vi "TSL_Sample.vi"() -> ()   [LabVIEW 2017]
uses:
  D:/test/FULLband-sts/Fullband_Sample/DLL/InstrumentDLL.dll
  DLL/InstrumentDLL.dll
  <vilib>/Utility/miscctls.llb/LVStringsAndValuesArrayTypeDef_DBL.ctl
  <vilib>/Utility/file.llb/Write To Spreadsheet File (DBL).vi
panel:
  in  "选项卡控件":T1(tab)
  in  "btnUsb_resouce":bool
  out "USB device number":string
  in  "Usb resouce":u16(ring)
  out "SweepSpeed Range":string
  in  "Port number":dbl
  in  "Target":enum32{"rdo550", "rdo570"}(radio)
  in  "btnSplit":bool
  out "GPIB Address":dbl
  out "GPIB Boad":dbl
  in  "btnGet_Visa":bool
  in  "Visa String":u16(ring)
  in  "Communication":T2(radio)
  in  "Terminator":enum32{"rdiCr", "rdiLf", "rdiCrLf"}(radio)
  out "Serial":string
  out "Product":string
  out "F/ W Vesion":string
  out "Frequency range":string
  out "Wavelength range":string
  out "APC Limit(dBm)":string
  out "APC Limit(mW)":string
  out "ATT range":string
  in  "Btn_Connect":bool
  in  "Btn_DisConnect":bool
  in  "Address/Device number":string
  out "unit":enum16{"dBm", "mW", ""}(ring)=enum.""
  out "txtshutter":enum16{"Shutter_Open", "Shutter_Close", ""}(ring)=enum.""
  out "status":enum16{"Coh_OFF", "Coh_ON", ""}(ring)=enum.""
  out "mode":enum16{"ACC", "APC", ""}(ring)=enum.""
  out "txtlds":enum16{"LD_OFF", "LD_ON", ""}(ring)=enum.""
  out "LAN Port number":i32
  in  "Get LAN Port":bool
  out "IP Address":string
  in  "Get IP Address":bool
  in  "BtnLD_ON":bool
  in  "BtnLD_OFF":bool
  in  "BtnCoh_ON":bool
  in  "BtnCoh_OFF":bool
  in  "BtnShutter_Open":bool
  in  "BtnShutter_Close":bool
  in  "BtnAPC":bool
  in  "BtnACC":bool
  in  "BtndBm":bool
  in  "BtnmW":bool
  in  "Setting ATT":dbl
  in  "Btn_SetATT":bool
  in  "Setting Power":dbl
  in  "Btn_SetdBm":bool
  in  "Btn_SetmW":bool
  in  "Btn_GetLD":bool
  in  "BtnPower_mode":bool
  in  "BtnCoh_Status":bool
  in  "BtnShutter_Status":bool
  in  "BtnUnit":bool
  out "txtreadatt":dbl
  in  "BtnAtt_value":bool
  out "txtreadpow":dbl
  in  "BtnPower_dBm":bool
  out "txtreadmw":dbl
  in  "BtnPower_mW":bool
  out "txtreadmoni":dbl
  in  "Btnmonitor_dBm":bool
  out "txtradmoni_mw":dbl
  in  "Btnmonitor_mW":bool
  in  "txtsetwave":dbl
  in  "Btn_SetWavelength":bool
  in  "txtsetfreq":dbl
  in  "Btn_SetFrequency":bool
  in  "txtsetft":dbl
  in  "Btn_SetFinetuning":bool
  in  "Btn_Wavelength":bool
  in  "Btn_Frequency":bool
  in  "Btn_Fine":bool
  out "txtwave":dbl
  out "txtfreq":dbl
  out "txtfine":dbl
  out "txtbusy":string
  in  "Btn_Busy":bool
  in  "Wait time(msec)":i32
  in  "Btn_Stangby":bool
  out "txttsl_err":string
  in  "Btn_error":bool
  out "Start mode":enum16{"Normal", "WaitingforTrigger", ""}(ring)=enum.""
  out "Trigger output":enum16{"None", "Stop", "Start", "Step", ""}(ring)=enum.""
  out "Trigger input":enum16{"Disable", "Enable", ""}(ring)=enum.""
  out "Sweep Mode":T3(ring)=enum.""
  out "txtg_sweep_su":T4(ring)=enum."Returning"
  out "Trigger Source":enum16{"Wavelength", "Time", ""}(ring)=enum.""
  in  "Speed(570)":u16(ring) caption="Speed(nm/sec)" items=["1"=1, "2"=2, "5"=5, "10"=10, "20"=20, "50"=50, "100"=100, "200"=200]
  in  "Speed":u16(ring)
  in  "Get speed table":bool
  in  "cmbTrigger_Source":enum16{"Wavelength", "Time", ""}(ring) caption="Trigger Source(570)"
  in  "txtstart":dbl caption="Start wavelength"
  in  "Btn_SetWavelength_Parameters":bool
  in  "txtstop":dbl caption="Stop wavelength"
  in  "txtstep":dbl=0.1 caption="Trigger/wave step"
  in  "txtspeed(550)":dbl caption="Speed(nm/sec)"
  in  "Btn_Other":bool
  in  "txtdelay":dbl caption="Delay time(sec)"
  in  "txtcycle":i32=1 caption="cycle"
  in  "cmbsm":T5(ring) caption="Sweep Mode"
  in  "cmbst_mod":enum16{"Disable", "Enable"}(ring) caption="Trigger input"
  in  "cmbtout":enum16{"None", "Stop", "Start", "Step"}(ring) caption="Trigger output"
  in  "cmbtin":enum16{"Normal", "Waiting for Trigger"}(ring) caption="Start mode"
  out "Start wavelength":dbl
  out "Stop wavelength":dbl
  out "Wavelength step":dbl
  out "Trigger step":dbl
  out "Speed(nm/sec)":dbl
  out "Delay time(sec)":dbl
  out "cycle":i32
  in  "BtnGet_setting":bool
  in  "Status":u16(ring) items=["Standby", "Running", "Pauseing", "WaitingforTrigger", "Returning"]
  in  "Wait time(msec)":i32
  in  "Btn_Waiting":bool
  in  "Btn_Status":bool
  in  "Btn_Minstep":bool
  in  "txtspeed":dbl=100.0
  out "txtcurrentc":i32
  in  "Btn_Current":bool
  in  "Btn_Start":bool
  in  "Btn_Stop":bool
  in  "Btn_SoftwareTrigger":bool
  in  "Btn_Pause":bool
  in  "Btn_ReStart":bool
  in  "Btn_GetLogg":bool
  out "TSL":refnum<k24>
  # "0. Connect Tool"
  # "1. Connect"
  # "Information"
  # "Power Control"
  # "Power status"
  # "Wavelength Control"
  # "Wavelength Status"
  # "Common Function"
  # "Sweep Setting"
  # "Other"
  # "Wavelength parameters"
  # "Other parameters"
  # "Sweep Speed(nm/s)"
  # "Sweep setting status"
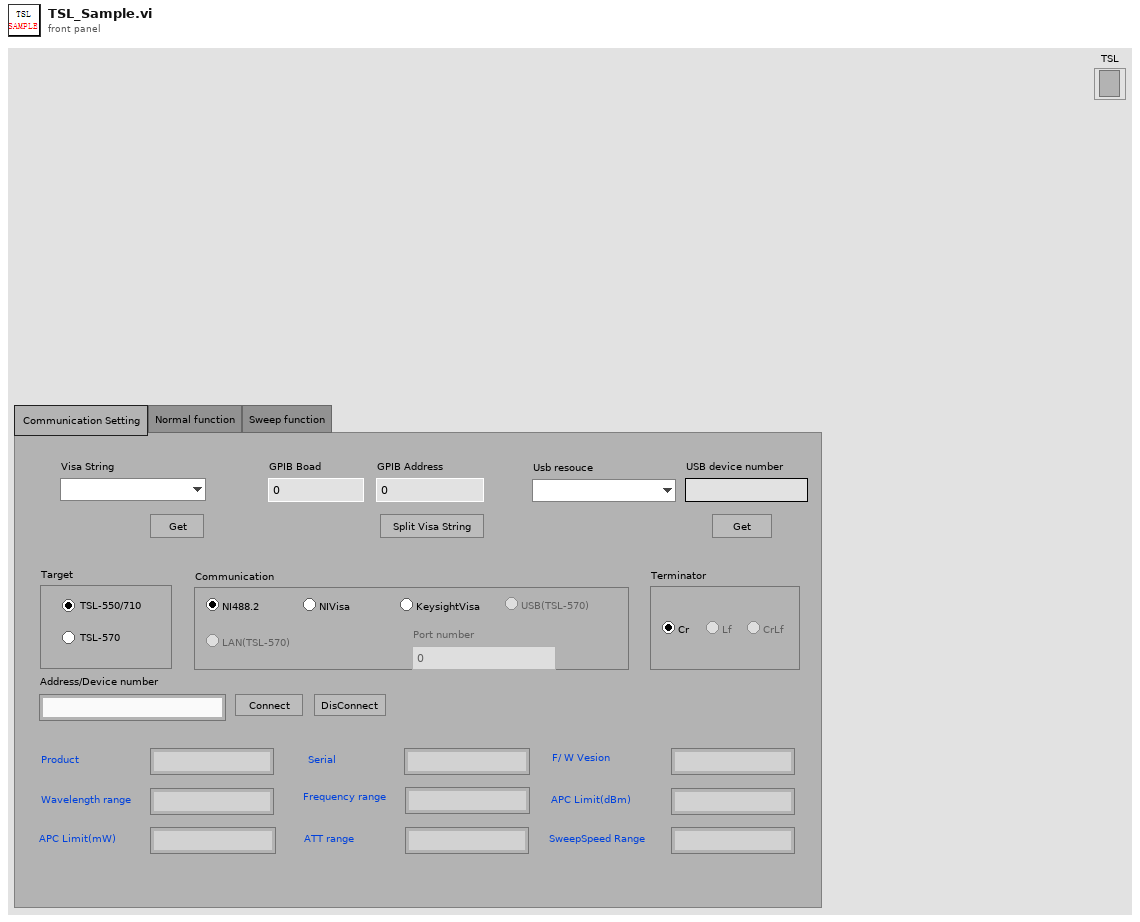
[diagram p1: front panel]
types:
  T1 = enum32{"Communication Setting ", "Normal function", "Sweep function"}
  T2 = enum32{"rdiNI488", "rdiNIvisa", "rdikysightvisa", "rdiUSB", "rdiLAN"}
  T3 = enum16{"Step_Oneway", "Continuous_Oneway", "Step_Twoway", "Continuous_Twoway", ""}
  T4 = enum16{"Standby", "Running", "Pausing", "WaitingforTrigger", "Returning"}
  T5 = enum16{"Step one way", "Continuous one way", "Step round trip", "Continuous round trip"}
  T6 = enum16{"Standby", "Running", "Pausing", "WaitingforTrigger", "Returning", ""}
  T7 = enum8{"Enabled", "Disabled", "Disabled and Grayed Out"}
  T8 = typedef "LVStringsAndValuesArrayTypeDef_DBL.ctl" = cluster{"String":string, "Value":dbl}[]
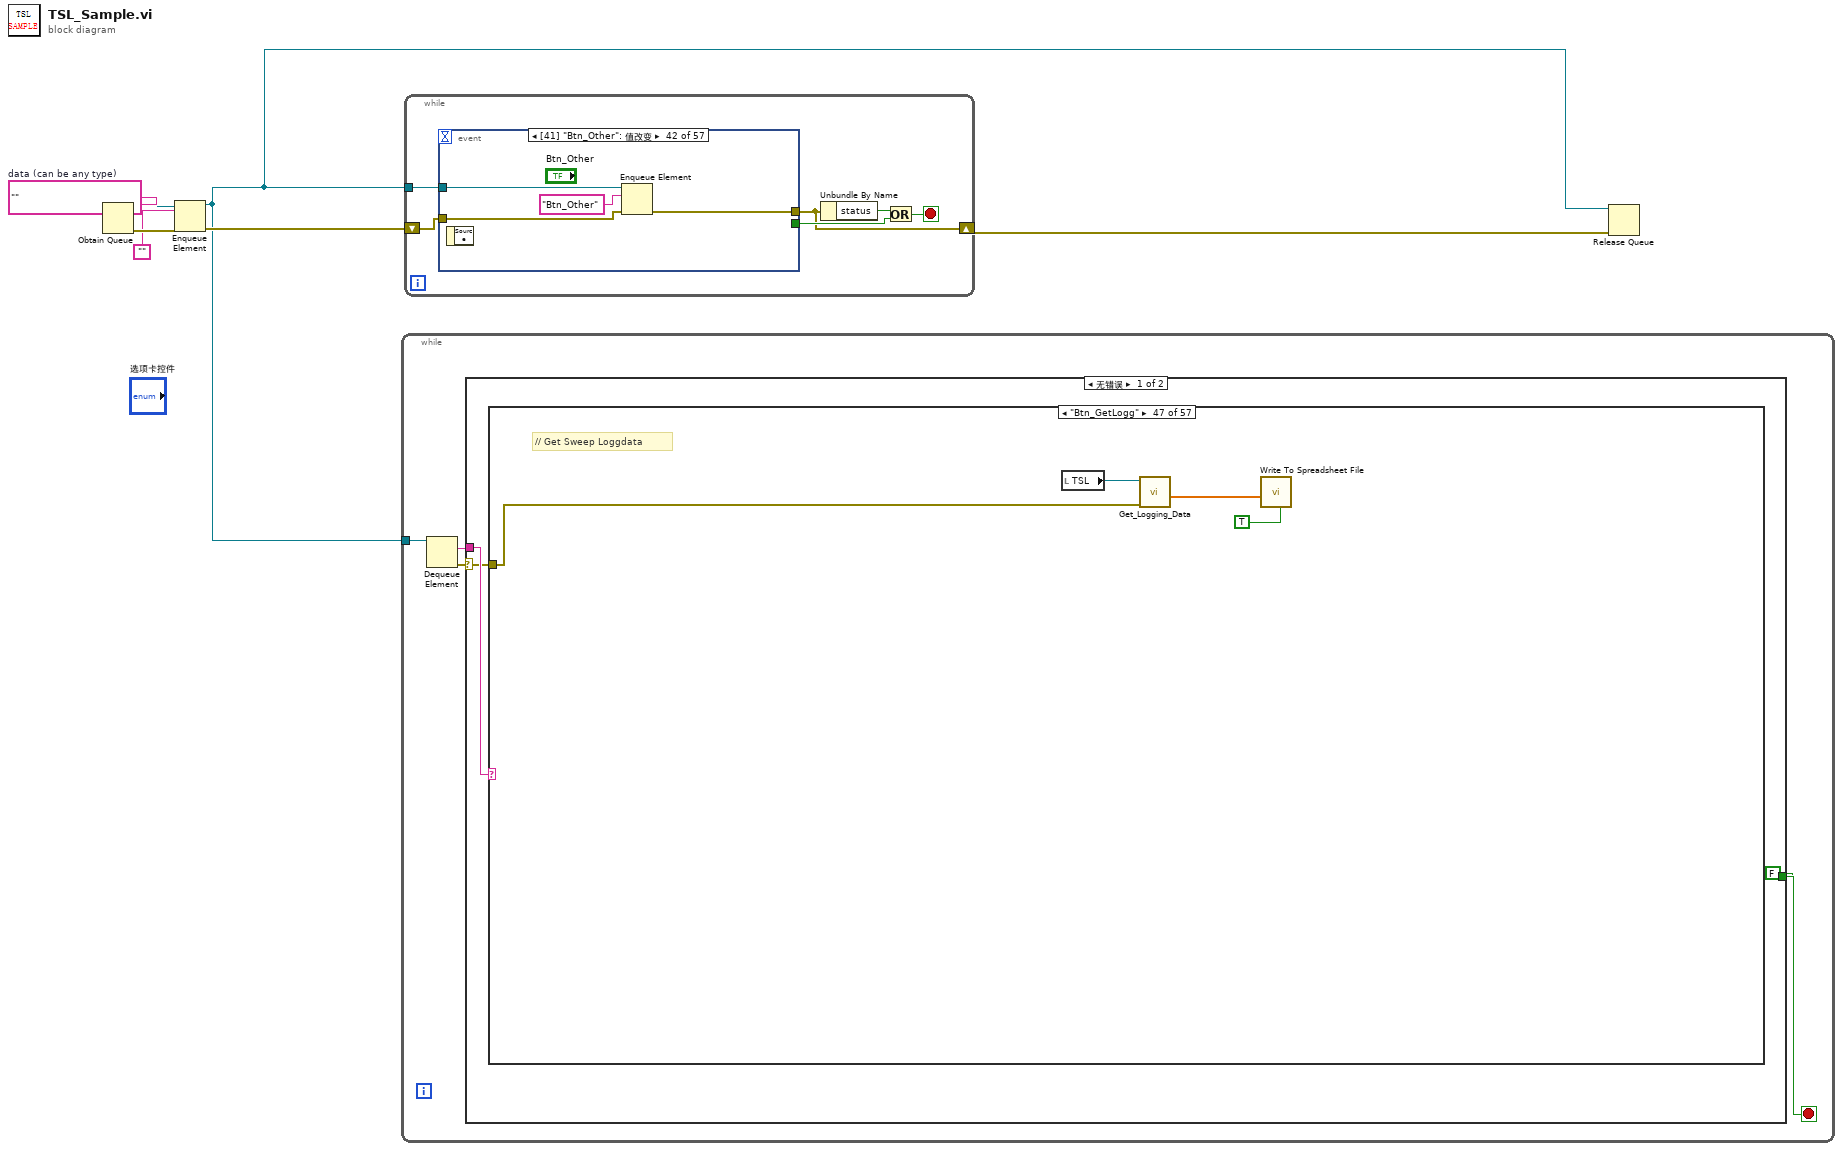
[diagram p0: block diagram]
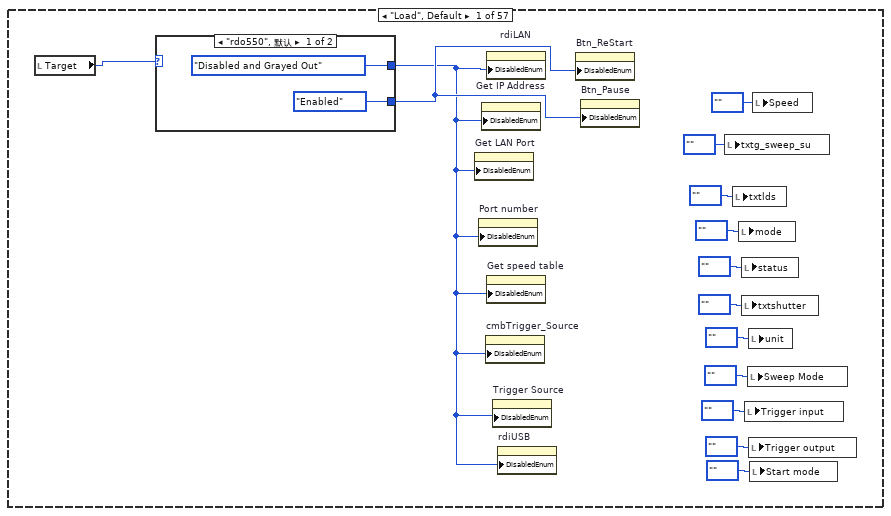
[diagram p2: hidden frame]
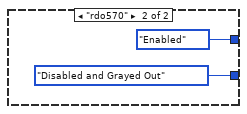
[diagram p3: hidden frame]
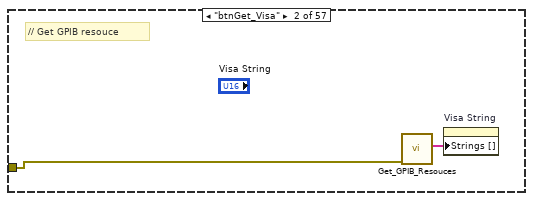
[diagram p4: hidden frame]
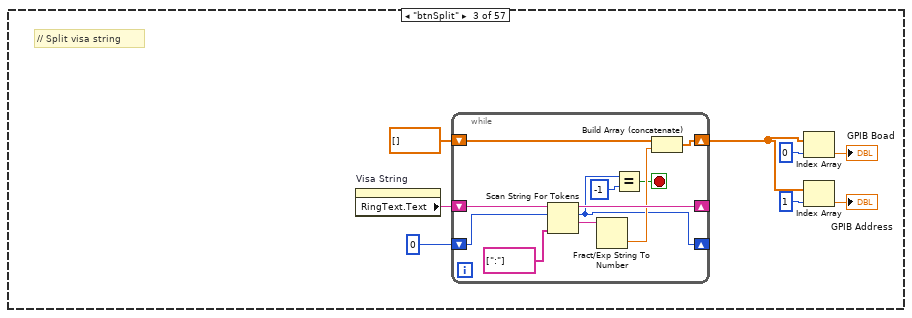
[diagram p5: hidden frame]
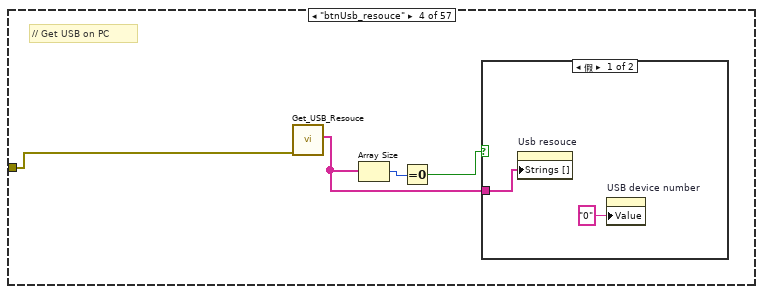
[diagram p6: hidden frame]
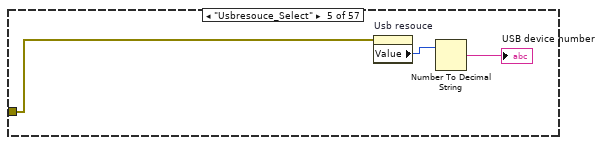
[diagram p8: hidden frame]
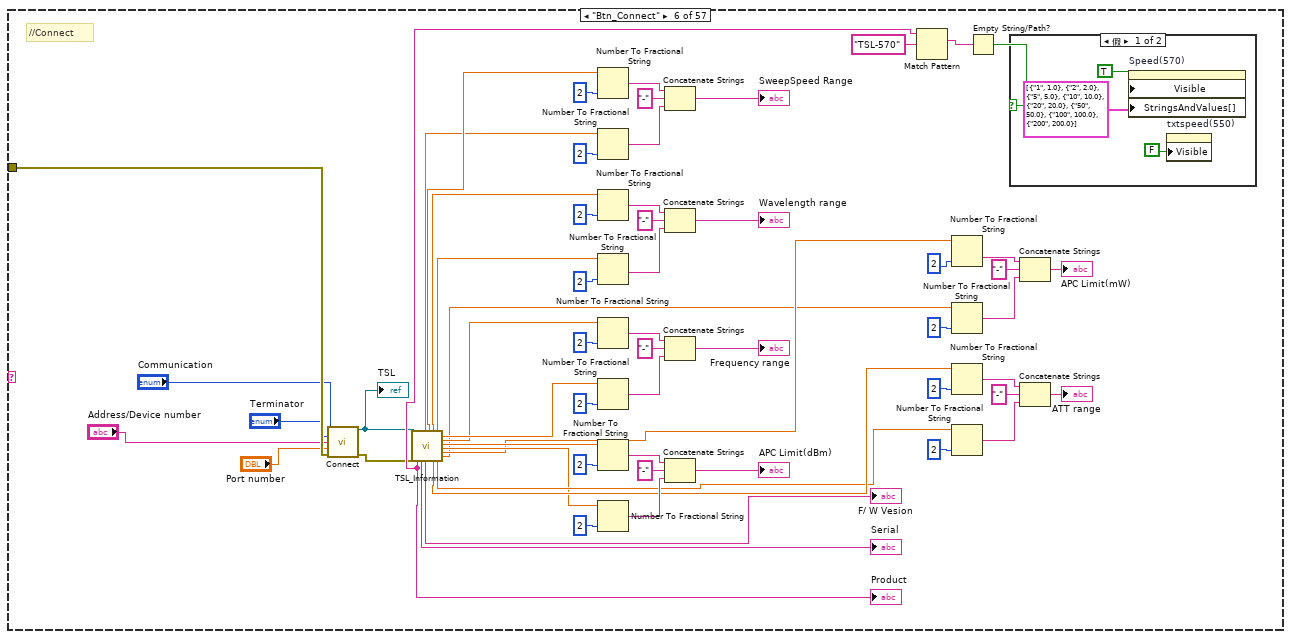
[diagram p9: hidden frame]
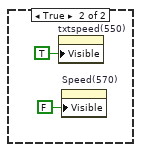
[diagram p10: hidden frame]
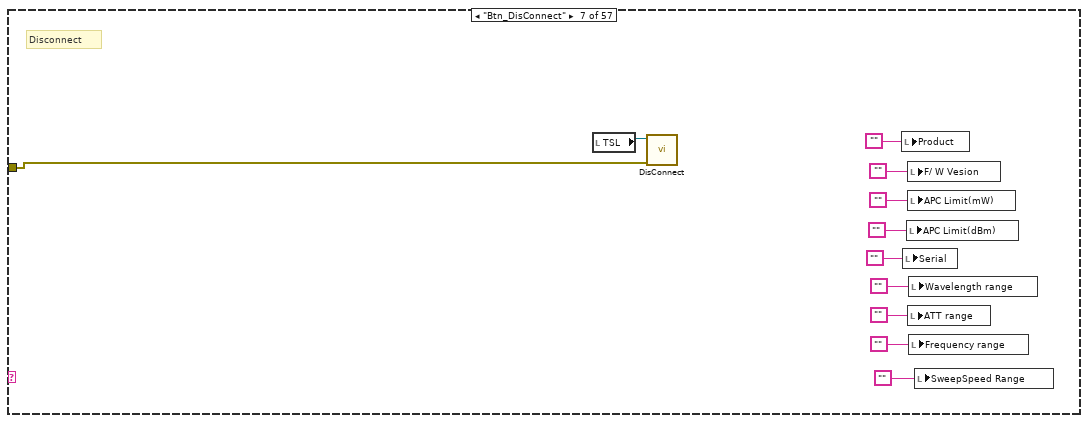
[diagram p11: hidden frame]
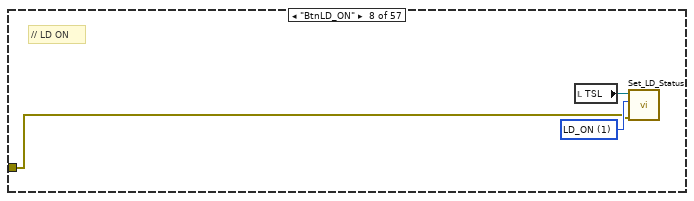
[diagram p12: hidden frame]
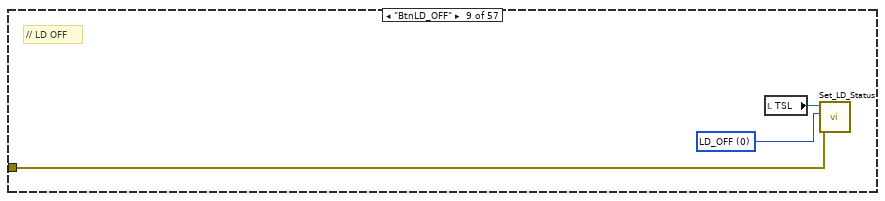
[diagram p13: hidden frame]
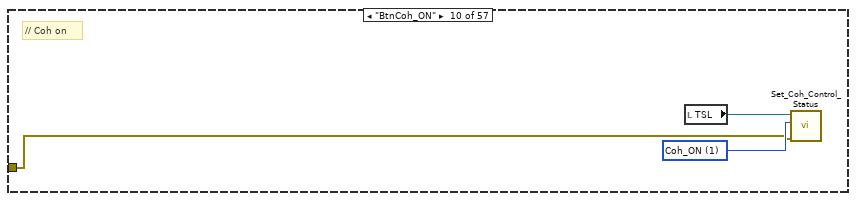
[diagram p14: hidden frame]
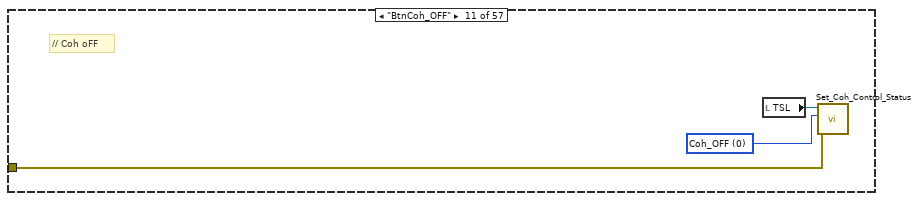
[diagram p15: hidden frame]
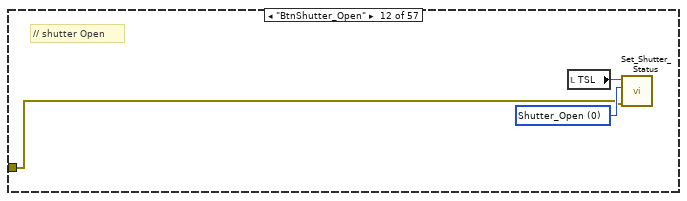
[diagram p16: hidden frame]
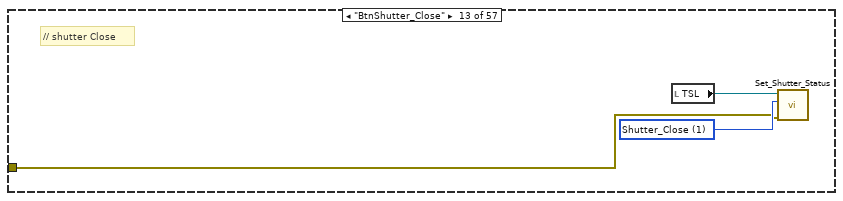
[diagram p17: hidden frame]
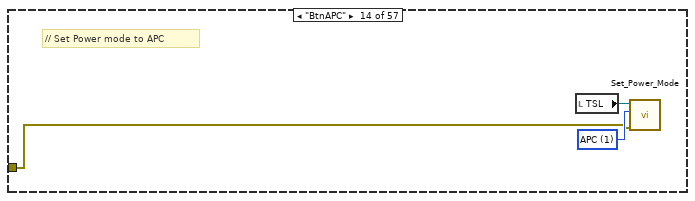
[diagram p18: hidden frame]
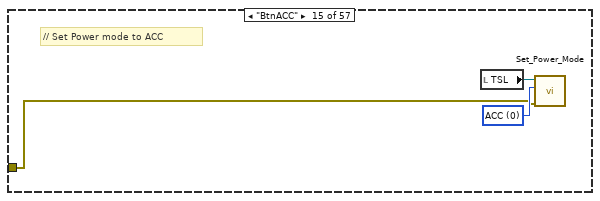
[diagram p19: hidden frame]
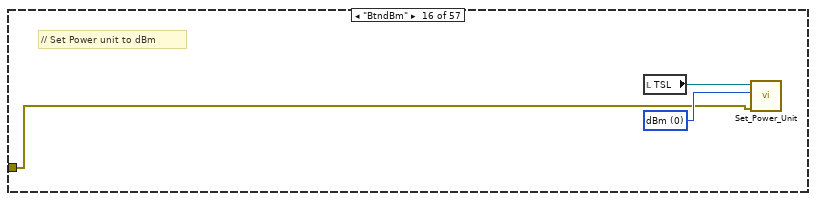
[diagram p20: hidden frame]
diagram:
  w4 = ""  # data (can be any type)
  n1 = Obtain Queue(element data type=w4) -> (queue out=w3:refnum<queue>, error out=w7:errorcluster)  [unwired: 4 in, 1 out]
  n2 = Enqueue Element(queue=w3, element="", error in (no error)=w7) -> (queue out=w1:refnum<queue>, error out=w6:errorcluster)  [unwired: 1 in, 1 out]
  n3 = while {
    tunnel: w1 -> [w11]
    stop <- w8 stop-if-true
    n4 = Dequeue Element(queue=w11) -> (element=w9:string, error out=w10:errorcluster)  [unwired: 2 in, 2 out]
    n5 = case shown="无错误" w10 {
      selector: w10 -> [w12 _]
      tunnel: w9 -> [w14 _]
      tunnel: [FALSE TRUE] -> w8
      frame No Error {
        n6 = case shown="\"Btn_GetLogg\"" w14 {
          tunnel: w12 -> [_ w33 _ w54 w62 w68 w129 w140 w143 w146 w149 w152 w155 w158 w161 w164 w167 w170 w173 w177 w179 w182 w185 w188 w191 w194 w197 w202 w215 _ w234 w238 w240 w244 w247 w250 w252 w255 w258 w261 w264 w267 w276 w300 w336 w351 w354 w357 w360 w368 w370 w372 w374 w378 w380 w383 _]
          frame "Load", Default {
            n7 = local read "Target"() -> (w27:enum32{"rdo550", "rdo570"})
            n8 = case shown="\"rdo550\", 默认" w27 {
              tunnel: [T7."Disabled and Grayed Out" ("禁用") T7."Enabled" ("禁用")] -> w26
              tunnel: [T7."Enabled" ("禁用") T7."Disabled and Grayed Out" ("禁用")] -> w28
              frame "rdo550", Default {
              }
              frame "rdo570" {
              }
            }
            n9 = property on="Get LAN Port" class="Bool"("DisabledEnum"=w26) -> ()  [unwired: 2 in, 2 out]
            n10 = property on="Port number" class="DigNum (严格)"("DisabledEnum"=w26) -> ()  [unwired: 2 in, 2 out]
            n11 = property on="Get IP Address" class="Bool"("DisabledEnum"=w26) -> ()  [unwired: 2 in, 2 out]
            n12 = property on="cmbTrigger_Source" class="Enum (严格)"("DisabledEnum"=w26) -> ()  [unwired: 2 in, 2 out]
            n13 = property on="rdiLAN" class="Bool (严格)"("DisabledEnum"=w26) -> ()  [unwired: 2 in, 2 out]
            n14 = property on="Get speed table" class="Bool"("DisabledEnum"=w26) -> ()  [unwired: 2 in, 2 out]
            n15 = property on="Trigger Source" class="Enum (严格)"("DisabledEnum"=w26) -> ()  [unwired: 2 in, 2 out]
            n16 = property on="rdiUSB" class="Bool (严格)"("DisabledEnum"=w26) -> ()  [unwired: 2 in, 2 out]
            n17 = property on="Btn_ReStart" class="Bool"("DisabledEnum"=w28) -> ()  [unwired: 2 in, 2 out]
            n18 = property on="Btn_Pause" class="Bool"("DisabledEnum"=w28) -> ()  [unwired: 2 in, 2 out]
            n19 = local write "txtg_sweep_su"(T6."" ("txtg_sweep_su")) -> ()
            n20 = local write "txtlds"(enum16{"LD_OFF", "LD_ON", ""}."" ("txtlds")) -> ()
            n21 = local write "mode"(enum16{"ACC", "APC", ""}."" ("mode")) -> ()
            n22 = local write "status"(enum16{"Coh_OFF", "Coh_ON", ""}."" ("status")) -> ()
            n23 = local write "txtshutter"(enum16{"Shutter_Open", "Shutter_Close", ""}."" ("txtshutter")) -> ()
            n24 = local write "Trigger input"(enum16{"Disable", "Enable", ""}."" ("Trigger input")) -> ()
            n25 = local write "Sweep Mode"(T3."" ("Sweep Mode")) -> ()
            n26 = local write "unit"(enum16{"dBm", "mW", ""}."" ("unit")) -> ()
            n27 = local write "Trigger output"(enum16{"None", "Stop", "Start", "Step", ""}."" ("Trigger output")) -> ()
            n28 = local write "Start mode"(enum16{"Normal", "WaitingforTrigger", ""}."" ("Start mode")) -> ()
            n29 = local write "Speed"(enum16{""}."" ("Speed")) -> ()
          }
          frame "btnGet_Visa" {
            # "// Get GPIB resouce"
            n30 = call "Get_GPIB_Resouces.vi"("error in (no error)"=w33) -> ("Get_GPIB_Resources"=w34:string[])  [unwired: 8 in, 2 out]
            n31 = property on="Visa String" class="Ring (严格)"("Strings []"=w34) -> ()  [unwired: 2 in, 2 out]
          }
          frame "btnSplit" {
            # "// Split visa string"
            n32 = property on="Visa String" class="Ring (严格)"() -> ("RingText.Text"=w38:string)  [unwired: 2 in, 2 out]
            n33 = while {
              shift-right: [w52] -> _
              shift-left: w38 -> [w53]
              shift-right: [w48] -> w40
              shift-left: dbl[] [] ("数组") -> [w49]
              shift-right: [w43] -> _
              shift-left: 0 ("偏移量") -> [w44]
              stop <- w46 stop-if-true
              n34 = Scan String For Tokens(6:string[] [":"] ("分隔符(\\s,\\t,\\r,\\n)"), 8:w44, 9:w53) -> (1:w51:string, 2:w43:i32, 3:w52:string)  [unwired: 3 in, 1 out]
              n35 = Fract/Exp String To Number(string=w51) -> (number=w50:dbl)  [unwired: 3 in, 1 out]
              n36 = Equal?(x=w43, y=-1) -> (x = y?=w46:bool)
              n37 = Build Array (concatenate)(w49, w50) -> (w48:dbl[])
            }
            n38 = Index Array(array=w40, index=0 ("索引")) -> (element=→"GPIB Boad":dbl)
            n39 = Index Array(array=w40, index=1 ("索引")) -> (element=→"GPIB Address":dbl)
          }
          frame "btnUsb_resouce" {
            # "// Get USB on PC"
            n40 = call "Get_USB_Resouce.vi"("error in (no error)"=w54) -> ("Get_USB_Resouce"=w55:string[])  [unwired: 8 in, 2 out]
            n41 = Array Size(array=w55) -> (size(s)=w57:i32)
            n42 = Equal To 0?(x=w57) -> (x = 0?=w56:bool)
            n43 = case shown="假" w56 {
              tunnel: w55 -> [w59 _]
              frame False {
                n44 = property on="Usb resouce" class="Ring (严格)"("Strings []"=w59) -> ()  [unwired: 2 in, 2 out]
                n45 = property on="USB device number" class="Str"("Value"="0" ("USB device number")) -> ()  [unwired: 2 in, 2 out]
              }
              frame True {
              }
            }
          }
          frame "Usbresouce_Select" {
            n46 = property on="Usb resouce" class="Ring (严格)"(error in=w62) -> ("Value"=w61:u16)  [unwired: 1 in, 2 out]
            n47 = Number To Decimal String(number=w61) -> (decimal integer string=→"USB device number":string)  [unwired: 1 in]
          }
          frame "Btn_Connect" {
            # "//Connect"
            n48 = call "Connect.vi"("Communication"="Communication", "Terminator"="Terminator", "Address/Device number"="Address/Device number", "Port"="Port number", "error in (no error)"=w68) -> ("Reference out"=w69:refnum<k24>, "error out"=w67:errorcluster)  [unwired: 9 in]
            "TSL" <- w69
            n49 = call "TSL_Information.vi"(".NET Reference in"=w69, "error in (no error)"=w67) -> ("ProductName"=w70:string, "SerialNumber"=→"Serial":string, "MaximumSpeed"=w79:dbl, "FWversion"=→"F/ W Vesion":string, "MinimumSpeed"=w80:dbl, "MinimunWavelength"=w78:dbl, "MinimumATTValue"=w82:dbl, "MaximumWavelength"=w77:dbl, "MaximumATTValue"=w81:dbl, "MaximumFrequency"=w76:dbl, "MinimunFrequency"=w75:dbl, "MinimumAPCPower_dBm"=w74:dbl, "MaximumAPCPower_dBm"=w73:dbl, "MinimumAPCPower_mW"=w72:dbl, "MaximumAPCPower_mW"=w71:dbl)  [unwired: 9 in, 2 out]
            "Product" <- w70
            n50 = Number To Fractional String(number=w80, precision (6)=i16 2 ("精度(6)")) -> (F-format string=w92:string)  [unwired: 2 in]
            n51 = Number To Fractional String(number=w79, precision (6)=i16 2 ("精度(6)")) -> (F-format string=w91:string)  [unwired: 2 in]
            n52 = Number To Fractional String(number=w78, precision (6)=i16 2 ("精度(6)")) -> (F-format string=w118:string)  [unwired: 2 in]
            n53 = Number To Fractional String(number=w77, precision (6)=i16 2 ("精度(6)")) -> (F-format string=w119:string)  [unwired: 2 in]
            n54 = Number To Fractional String(number=w75, precision (6)=i16 2 ("精度(6)")) -> (F-format string=w123:string)  [unwired: 2 in]
            n55 = Number To Fractional String(number=w76, precision (6)=i16 2 ("精度(6)")) -> (F-format string=w122:string)  [unwired: 2 in]
            n56 = Number To Fractional String(number=w74, precision (6)=i16 2 ("精度(6)")) -> (F-format string=w114:string)  [unwired: 2 in]
            n57 = Number To Fractional String(number=w73, precision (6)=i16 2 ("精度(6)")) -> (F-format string=w113:string)  [unwired: 2 in]
            n58 = Concatenate Strings(w92, "-" ("字符串"), w91) -> (→"SweepSpeed Range":string)
            n59 = Concatenate Strings(w118, "-" ("字符串"), w119) -> (→"Wavelength range":string)
            n60 = Concatenate Strings(w123, "-" ("字符串"), w122) -> (→"Frequency range":string)
            n61 = Concatenate Strings(w114, "-" ("字符串"), w113) -> (→"APC Limit(dBm)":string)
            n62 = Match Pattern(string=w70, regular expression="TSL-570" ("正则表达式")) -> (match substring=w86:string)  [unwired: 1 in, 3 out]
            n63 = Number To Fractional String(number=w72, precision (6)=i16 2 ("精度(6)")) -> (F-format string=w111:string)  [unwired: 2 in]
            n64 = Number To Fractional String(number=w71, precision (6)=i16 2 ("精度(6)")) -> (F-format string=w110:string)  [unwired: 2 in]
            n65 = Number To Fractional String(number=w82, precision (6)=i16 2 ("精度(6)")) -> (F-format string=w116:string)  [unwired: 2 in]
            n66 = Number To Fractional String(number=w81, precision (6)=i16 2 ("精度(6)")) -> (F-format string=w115:string)  [unwired: 2 in]
            n67 = Empty String/Path?(string/path=w86) -> (empty?=w85:bool)
            n68 = case shown="假" w85 {
              frame False {
                n69 = property on="Speed(570)" class="Ring (严格)"("Visible"=TRUE ("可见"), "StringsAndValues[]"=T8 [{"String"="1", "Value"=1.0}, {"String"="2", "Value"=2.0}, {"String"="5", "Value"=5.0}, {"String"="10", "Value"=10.0}, {"String"="20", "Value"=20.0}, {"String"="50", "Value"=50.0}, {"String"="100", "Value"=100.0}, {"String"="200", "Value"=200.0}] ("Strings And Values []")) -> ()  [unwired: 2 in, 2 out]
                n70 = property on="txtspeed(550)" class="DigNum (严格)"("Visible"=FALSE ("可见")) -> ()  [unwired: 2 in, 2 out]
              }
              frame True {
                n71 = property on="txtspeed(550)" class="DigNum (严格)"("Visible"=TRUE ("可见")) -> ()  [unwired: 2 in, 2 out]
                n72 = property on="Speed(570)" class="Ring (严格)"("Visible"=FALSE ("可见")) -> ()  [unwired: 2 in, 2 out]
              }
            }
            n73 = Concatenate Strings(w111, "-" ("字符串"), w110) -> (→"APC Limit(mW)":string)
            n74 = Concatenate Strings(w116, "-" ("字符串"), w115) -> (→"ATT range":string)
          }
          frame "Btn_DisConnect" {
            # "Disconnect"
            n75 = local read "TSL"() -> (w131:refnum<k24>)
            n76 = call "DisConnect.vi"("error in (no error)"=w129, ".NET Reference in"=w131) -> ()  [unwired: 4 in, 2 out]
            n77 = local write "Product"("") -> ()
            n78 = local write "Serial"("") -> ()
            n79 = local write "APC Limit(dBm)"("") -> ()
            n80 = local write "F/ W Vesion"("") -> ()
            n81 = local write "APC Limit(mW)"("") -> ()
            n82 = local write "ATT range"("") -> ()
            n83 = local write "Wavelength range"("") -> ()
            n84 = local write "Frequency range"("") -> ()
            n85 = local write "SweepSpeed Range"("") -> ()
          }
          frame "BtnLD_ON" {
            w142 = 1 items=["LD_OFF", "LD_ON"] ("status 2")
            # "// LD ON"
            n86 = local read "TSL"() -> (w141:refnum<k24>)
            n87 = call "Set_LD_Status.vi"("error in (no error)"=w140, "status"=w142, ".NET Reference in"=w141) -> ()  [unwired: 7 in, 2 out]
          }
          frame "BtnLD_OFF" {
            w144 = 0 items=["LD_OFF", "LD_ON"] ("status 2")
            # "// LD OFF"
            n88 = local read "TSL"() -> (w145:refnum<k24>)
            n89 = call "Set_LD_Status.vi"("error in (no error)"=w143, "status"=w144, ".NET Reference in"=w145) -> ()  [unwired: 7 in, 2 out]
          }
          frame "BtnCoh_ON" {
            w147 = 1 items=["Coh_OFF", "Coh_ON"] ("status 2")
            # "// Coh on"
            n90 = local read "TSL"() -> (w148:refnum<k24>)
            n91 = call "Set_Coh_Control_Status.vi"(".NET Reference in"=w148, "status"=w147, "error in (no error)"=w146) -> ()  [unwired: 6 in, 2 out]
          }
          frame "BtnCoh_OFF" {
            w150 = 0 items=["Coh_OFF", "Coh_ON"] ("status 2")
            # "// Coh oFF"
            n92 = local read "TSL"() -> (w151:refnum<k24>)
            n93 = call "Set_Coh_Control_Status.vi"(".NET Reference in"=w151, "status"=w150, "error in (no error)"=w149) -> ()  [unwired: 6 in, 2 out]
          }
          frame "BtnShutter_Open" {
            w153 = 0 items=["Shutter_Open", "Shutter_Close"] ("status 2")
            # "// shutter Open"
            n94 = local read "TSL"() -> (w154:refnum<k24>)
            n95 = call "Set_Shutter_Status.vi"(".NET Reference in"=w154, "status"=w153, "error in (no error)"=w152) -> ()  [unwired: 6 in, 2 out]
          }
          frame "BtnShutter_Close" {
            w156 = 1 items=["Shutter_Open", "Shutter_Close"] ("status 2")
            # "// shutter Close"
            n96 = local read "TSL"() -> (w157:refnum<k24>)
            n97 = call "Set_Shutter_Status.vi"(".NET Reference in"=w157, "status"=w156, "error in (no error)"=w155) -> ()  [unwired: 6 in, 2 out]
          }
          frame "BtnAPC" {
            w159 = 1 items=["ACC", "APC"] ("mode")
            # "// Set Power mode to APC"
            n98 = local read "TSL"() -> (w160:refnum<k24>)
            n99 = call "Set_Power_Mode.vi"(".NET Reference in"=w160, "mode"=w159, "error in (no error)"=w158) -> ()  [unwired: 6 in, 2 out]
          }
          frame "BtnACC" {
            w162 = 0 items=["ACC", "APC"] ("mode")
            # "// Set Power mode to ACC"
            n100 = local read "TSL"() -> (w163:refnum<k24>)
            n101 = call "Set_Power_Mode.vi"(".NET Reference in"=w163, "mode"=w162, "error in (no error)"=w161) -> ()  [unwired: 6 in, 2 out]
          }
          frame "BtndBm" {
            w165 = 0 items=["dBm", "mW"] ("unit")
            # "// Set Power unit to dBm"
            n102 = local read "TSL"() -> (w166:refnum<k24>)
            n103 = call "Set_Power_Unit.vi"(".NET Reference in"=w166, "unit"=w165, "error in (no error)"=w164) -> ()  [unwired: 6 in, 2 out]
          }
          frame "BtnmW" {
            w168 = 1 items=["dBm", "mW"] ("unit")
            # "// Set Power unit to mW"
            n104 = local read "TSL"() -> (w169:refnum<k24>)
            n105 = call "Set_Power_Unit.vi"(".NET Reference in"=w169, "unit"=w168, "error in (no error)"=w167) -> ()  [unwired: 6 in, 2 out]
          }
          frame "Btn_SetATT" {
            # "// SetATT"
            n106 = local read "TSL"() -> (w172:refnum<k24>)
            n107 = call "Set_Att_Value.vi"(".NET Reference in"=w172, "Setting ATT"="Setting ATT", "error in (no error)"=w170) -> ()  [unwired: 5 in, 2 out]
          }
          frame "Btn_SetdBm" {
            # "// Set Power dBm"
            n108 = local read "TSL"() -> (w175:refnum<k24>)
            n109 = call "Set_APC_Power_dBm.vi"(".NET Reference in"=w175, "Setting Power"="Setting Power", "error in (no error)"=w173) -> ()  [unwired: 6 in, 2 out]
          }
          frame "Btn_SetmW" {
            # "// Set Power mW"
            n110 = local read "Setting Power"() -> (w176:dbl)
            n111 = local read "TSL"() -> (w178:refnum<k24>)
            n112 = call "Set_APC_Power_mW.vi"(".NET Reference in"=w178, "Setting Power"=w176, "error in (no error)"=w177) -> ()  [unwired: 6 in, 2 out]
          }
          frame "Btn_SetWavelength" {
            # "// set Wavelength"
            n113 = local read "TSL"() -> (w181:refnum<k24>)
            n114 = call "Set_Wavelength.vi"("error in (no error)"=w179, "txtsetwave"="txtsetwave", ".NET Reference in"=w181) -> ()  [unwired: 3 in, 2 out]
          }
          frame "Btn_SetFrequency" {
            # "// set Frequency"
            n115 = local read "TSL"() -> (w184:refnum<k24>)
            n116 = call "Set_Frequency.vi"("error in (no error)"=w182, "txtsetfreq"="txtsetfreq", ".NET Reference in"=w184) -> ()  [unwired: 7 in, 2 out]
          }
          frame "Btn_SetFinetuning" {
            # "// Set Finetuning"
            n117 = local read "TSL"() -> (w187:refnum<k24>)
            n118 = call "Set_Finetuning.vi"("error in (no error)"=w185, "txtsetft"="txtsetft", ".NET Reference in"=w187) -> ()  [unwired: 7 in, 2 out]
          }
          frame "Btn_Wavelength" {
            # "// Get Setting Wavelength Value"
            n119 = local read "TSL"() -> (w189:refnum<k24>)
            n120 = call "Get_Wavelength.vi"("error in (no error)"=w188, ".NET Reference in"=w189) -> ("wav"=→"txtwave":dbl)  [unwired: 7 in, 2 out]
          }
          frame "Btn_Frequency" {
            # "// Get Setting Frequency"
            n121 = local read "TSL"() -> (w192:refnum<k24>)
            n122 = call "Get_Frequency.vi"("error in (no error)"=w191, ".NET Reference in"=w192) -> ("freq"=→"txtfreq":dbl)  [unwired: 7 in, 2 out]
          }
          frame "Btn_Fine" {
            # "// Get Fine tuning value"
            n123 = local read "TSL"() -> (w195:refnum<k24>)
            n124 = call "Get_Finetuning.vi"("error in (no error)"=w194, ".NET Reference in"=w195) -> ("ftval"=→"txtfine":dbl)  [unwired: 7 in, 2 out]
          }
          frame "Btn_Busy" {
            # "// Get Busy status"
            n125 = local read "TSL"() -> (w199:refnum<k24>)
            n126 = call "Get_Busy_Status.vi"("error in (no error)"=w197, ".NET Reference in"=w199) -> ("busyflag"=w198:bool)  [unwired: 7 in, 2 out]
            n127 = case shown="真" w198 {
              frame False {
                n128 = local write "txtbusy"("Standby") -> ()
              }
              frame True {
                "txtbusy" <- "Busy"
              }
            }
          }
          frame "Btn_Stangby" {
            # "// Waiting for standby until wait time"
            n129 = flat-sequence {
              tunnel: [w210] -> w204
              tunnel: w202 -> [w212]
              tunnel: [w214] -> w203
              frame #0 {
                n130 = Tick Count (ms)() -> (millisecond timer value=w210:u32)
              }
              frame #1 {
                n131 = local read "TSL"() -> (w213:refnum<k24>)
                n132 = call "TSL_Busy_Check.vi"("error in (no error)"=w212, "Wait time(msec)"="Wait time(msec)", ".NET Reference in"=w213) -> ()  [unwired: 7 in, 2 out]
              }
              frame #2 {
                n133 = Tick Count (ms)() -> (millisecond timer value=w214:u32)
              }
            }
            n134 = Subtract(x=w203, y=w204) -> (x-y=w205:u32)
            n135 = Number To Decimal String(number=w205) -> (decimal integer string=w208:string)  [unwired: 1 in]
            n136 = Concatenate Strings("Busy time :", w208, "ms") -> (w206:string)
            n137 = One Button Dialog(message=w206) -> ()  [unwired: 1 in, 1 out]
          }
          frame "Get speed table" {
            n138 = local read "Target"() -> (w216:enum32{"rdo550", "rdo570"})
            n139 = case shown="\"rdo570\"" w216 {
              tunnel: w215 -> [_ w219]
              frame "rdo550", Default {
              }
              frame "rdo570" {
                n140 = local read "TSL"() -> (w222:refnum<k24>)
                n141 = call "Get_Sweep_Speed_table.vi"("error in (no error)"=w219, ".NET Reference in"=w222) -> ("error out"=w218:errorcluster, "Get_Sweep_Speed_table"=w221:dbl[])  [unwired: 7 in, 1 out]
                n142 = for {
                  tunnel: w221 -> [w226] mode=indexing
                  shift-right: [w223] -> w217
                  shift-left: string[] [] ("添加的数组") -> [w224]
                  n143 = Number To Decimal String(number=w226) -> (decimal integer string=w225:string)  [unwired: 1 in]
                  n144 = Build Array (concatenate)(w224, w225) -> (w223:string[])
                }
                n145 = property on="Speed" class="Ring (严格)"(error in=w218, "Strings []"=w217) -> ()  [unwired: 1 in, 2 out]
              }
            }
          }
          frame "Target" {
            n146 = case shown="\"rdo550\", 默认" "Target" {
              tunnel: [T7."Disabled and Grayed Out" ("禁用") T7."Enabled" ("禁用")] -> w227
              tunnel: [T7."Enabled" ("禁用") T7."Disabled and Grayed Out" ("禁用")] -> w229
              frame "rdo550", Default {
              }
              frame "rdo570" {
              }
            }
            n147 = property on="Get LAN Port" class="Bool"("DisabledEnum"=w227) -> ()  [unwired: 2 in, 2 out]
            n148 = property on="Port number" class="DigNum (严格)"("DisabledEnum"=w227) -> ()  [unwired: 2 in, 2 out]
            n149 = property on="Get IP Address" class="Bool"("DisabledEnum"=w227) -> ()  [unwired: 2 in, 2 out]
            n150 = property on="cmbTrigger_Source" class="Enum (严格)"("DisabledEnum"=w227) -> ()  [unwired: 2 in, 2 out]
            n151 = property on="rdiLAN" class="Bool (严格)"("DisabledEnum"=w227) -> ()  [unwired: 2 in, 2 out]
            n152 = property on="Get speed table" class="Bool"("DisabledEnum"=w227) -> ()  [unwired: 2 in, 2 out]
            n153 = property on="Trigger Source" class="Enum (严格)"("DisabledEnum"=w227) -> ()  [unwired: 2 in, 2 out]
            n154 = property on="rdiUSB" class="Bool (严格)"("DisabledEnum"=w227) -> ()  [unwired: 2 in, 2 out]
            n155 = property on="Btn_ReStart" class="Bool"("DisabledEnum"=w229) -> ()  [unwired: 2 in, 2 out]
            n156 = property on="Btn_Pause" class="Bool"("DisabledEnum"=w229) -> ()  [unwired: 2 in, 2 out]
          }
          frame "Btn_error" {
            # "// Get TSL error code"
            n157 = local read "TSL"() -> (w236:refnum<k24>)
            n158 = call "Get_System_Error.vi"("error in (no error)"=w234, ".NET Reference in"=w236) -> ("error"=→"txttsl_err":string)  [unwired: 7 in, 2 out]
          }
          frame "Btn_GetLD" {
            # "// Get LD Status"
            n159 = local read "TSL"() -> (w239:refnum<k24>)
            n160 = call "Get_LD_Status.vi"("error in (no error)"=w238, ".NET Reference in"=w239) -> ("status"=→"txtlds":enum16{"LD_OFF", "LD_ON", ""})  [unwired: 7 in, 2 out]
          }
          frame "BtnPower_mode" {
            # "// Get Power Mode"
            n161 = local read "TSL"() -> (w242:refnum<k24>)
            n162 = call "Get_Power_Mode.vi"("error in (no error)"=w240, ".NET Reference in"=w242) -> ("mode"=→"mode":enum16{"ACC", "APC", ""})  [unwired: 7 in, 2 out]
          }
          frame "BtnCoh_Status" {
            # "// Get coh Status"
            n163 = local read "TSL"() -> (w245:refnum<k24>)
            n164 = call "Get_Coh_Control_Status.vi"("error in (no error)"=w244, ".NET Reference in"=w245) -> ("status"=→"status":enum16{"Coh_OFF", "Coh_ON", ""})  [unwired: 7 in, 2 out]
          }
          frame "BtnShutter_Status" {
            # "// Get  shutter status"
            n165 = local read "TSL"() -> (w248:refnum<k24>)
            n166 = call "Get_Shutter_Status.vi"("error in (no error)"=w247, ".NET Reference in"=w248) -> ("status"=→"txtshutter":enum16{"Shutter_Open", "Shutter_Close", ""})  [unwired: 7 in, 2 out]
          }
          frame "BtnUnit" {
            # "// Get Unit"
            n167 = local read "TSL"() -> (w251:refnum<k24>)
            n168 = call "Get_Power_Unit.vi"("error in (no error)"=w250, ".NET Reference in"=w251) -> ("unit"=→"unit":enum16{"dBm", "mW", ""})  [unwired: 7 in, 2 out]
          }
          frame "BtnAtt_value" {
            # "// Get Att value"
            n169 = local read "TSL"() -> (w253:refnum<k24>)
            n170 = call "Get_Att_Value.vi"("error in (no error)"=w252, ".NET Reference in"=w253) -> ("att out"=→"txtreadatt":dbl)  [unwired: 7 in, 2 out]
          }
          frame "BtnPower_dBm" {
            # "// Get Setting power dBm"
            n171 = local read "TSL"() -> (w256:refnum<k24>)
            n172 = call "Get_Setting_Power_dBm.vi"("error in (no error)"=w255, ".NET Reference in"=w256) -> ("pow out"=→"txtreadpow":dbl)  [unwired: 7 in, 2 out]
          }
          frame "BtnPower_mW" {
            # "// Get Setting power mW"
            n173 = local read "TSL"() -> (w259:refnum<k24>)
            n174 = call "Get_Setting_Power_mW.vi"("error in (no error)"=w258, ".NET Reference in"=w259) -> ("pow out"=→"txtreadmw":dbl)  [unwired: 7 in, 2 out]
          }
          frame "Btnmonitor_dBm" {
            # "// Get Monitor power dBm"
            n175 = local read "TSL"() -> (w263:refnum<k24>)
            n176 = call "Get_Monitor_Power_dBm.vi"("error in (no error)"=w261, ".NET Reference in"=w263) -> ("power out"=→"txtreadmoni":dbl)  [unwired: 7 in, 2 out]
          }
          frame "Btnmonitor_mW" {
            (unwired) 0.0 ("pow")
            # "// Get Monitor power mW"
            n177 = local read "TSL"() -> (w266:refnum<k24>)
            n178 = call "Get_Monitor_Power_mW.vi"("error in (no error)"=w264, ".NET Reference in"=w266) -> ("pow out"=→"txtradmoni_mw":dbl)  [unwired: 7 in, 2 out]
          }
          frame "Btn_SetWavelength_Parameters" {
            # "// set Wavelength"
            n179 = local read "TSL"() -> (w275:refnum<k24>)
            n180 = call "Set_Sweep_Wavelength.vi"("error in (no error)"=w267, "Stop wavelength"="txtstop", "Start wavelength"="txtstart", ".NET Reference in"=w275) -> ("error out"=w268:errorcluster, ".NET Reference out"=w271:refnum<k24>)  [unwired: 6 in]
            n181 = call "Set_Wavelength_Step.vi"("error in (no error)"=w268, "wave step"="txtstep", ".NET Reference in"=w271) -> ("error out"=w269:errorcluster, ".NET Reference out"=w270:refnum<k24>)  [unwired: 7 in]
            n182 = call "Set_Trigger_Step.vi"("error in (no error)"=w269, "Trigger step"="txtstep", ".NET Reference in"=w270) -> ()  [unwired: 7 in, 2 out]
          }
          frame "Btn_Other" {
            # "// Set Sweep Parameters"
            n183 = local read "Target"() -> (w277:enum32{"rdo550", "rdo570"})
            n184 = case shown="\"rdo570\"" w277 {
              tunnel: ["txtspeed(550)" "Speed(570)"] -> w293
              frame "rdo550", Default {
              }
              frame "rdo570" {
              }
            }
            n185 = local read "TSL"() -> (w292:refnum<k24>)
            n186 = call "Set_Sweep_Speed.vi"("error in (no error)"=w276, "Speed(nm/sec)"=w293, ".NET Reference in"=w292) -> ("error out"=w280:errorcluster, ".NET Reference out"=w281:refnum<k24>)  [unwired: 7 in]
            n187 = call "Set_Sweep_Delay.vi"("error in (no error)"=w280, "Delay time(sec)"="txtdelay", ".NET Reference in"=w281) -> ("error out"=w282:errorcluster, ".NET Reference out"=w283:refnum<k24>)  [unwired: 7 in]
            n188 = call "Set_Sweep_Cycle.vi"("error in (no error)"=w282, "cycle"="txtcycle", ".NET Reference in"=w283) -> ("error out"=w284:errorcluster, ".NET Reference out"=w288:refnum<k24>)  [unwired: 7 in]
            n189 = call "Set_Sweep_Mode_Parameters.vi"("Start mode"="cmbtin", "Sweep Mode"="cmbsm", "error in (no error)"=w284, "Trigger input"="cmbst_mod", "Trigger output"="cmbtout", ".NET Reference in"=w288) -> ("error out"=w279:errorcluster, "Reference out"=w278:refnum<k24>)  [unwired: 4 in]
            n190 = case shown="\"rdo570\"" w277 {
              tunnel: w279 -> [_ w298]
              tunnel: w278 -> [_ w297]
              frame "rdo550", Default {
              }
              frame "rdo570" {
                n191 = call "Set_TriggerOutput_Source.vi"("error in (no error)"=w298, "mode"="cmbTrigger_Source", ".NET Reference in"=w297) -> ()  [unwired: 7 in, 2 out]
              }
            }
          }
          frame "BtnGet_setting" {
            # "// get sweep paremters"
            n192 = local read "TSL"() -> (w332:refnum<k24>)
            n193 = call "Get_Sweep_Mode.vi"("error in (no error)"=w300, ".NET Reference in"=w332) -> ("error out"=w329:errorcluster, "smod"=→"Sweep Mode":T3, ".NET Reference out"=w330:refnum<k24>)  [unwired: 7 in]
            n194 = call "Get_Input_Trigger_Mode.vi"("error in (no error)"=w329, ".NET Reference in"=w330) -> ("error out"=w305:errorcluster, "mode"=→"Trigger input":enum16{"Disable", "Enable", ""}, ".NET Reference out"=w304:refnum<k24>)  [unwired: 7 in]
            n195 = call "Get_Trigger_Output_Mode.vi"("error in (no error)"=w305, ".NET Reference in"=w304) -> ("error out"=w306:errorcluster, "mode"=→"Trigger output":enum16{"None", "Stop", "Start", "Step", ""}, ".NET Reference out"=w307:refnum<k24>)  [unwired: 7 in]
            n196 = call "Get_Sweep_Start_Mode.vi"("error in (no error)"=w306, ".NET Reference in"=w307) -> ("error out"=w309:errorcluster, "mode"=→"Start mode":enum16{"Normal", "WaitingforTrigger", ""}, ".NET Reference out"=w308:refnum<k24>)  [unwired: 7 in]
            n197 = call "Get_Sweep_Speed.vi"("error in (no error)"=w309, ".NET Reference in"=w308) -> ("error out"=w311:errorcluster, "speed out"=→"Speed(nm/sec)":dbl, ".NET Reference out"=w310:refnum<k24>)  [unwired: 7 in]
            n198 = call "Get_Sweep_Wavelength.vi"("error in (no error)"=w311, ".NET Reference in"=w310) -> ("error out"=w312:errorcluster, "endwave out"=→"Stop wavelength":dbl, "startwave out"=→"Start wavelength":dbl, ".NET Reference out"=w313:refnum<k24>)  [unwired: 6 in]
            n199 = call "Get_Sweep_Delay.vi"("error in (no error)"=w312, ".NET Reference in"=w313) -> ("error out"=w316:errorcluster, "delay out"=→"Delay time(sec)":dbl, ".NET Reference out"=w314:refnum<k24>)  [unwired: 7 in]
            n200 = call "Get_Sweep_Cycle.vi"("error in (no error)"=w316, ".NET Reference in"=w314) -> ("error out"=w317:errorcluster, "times out"=→"cycle":i32, ".NET Reference out"=w315:refnum<k24>)  [unwired: 7 in]
            n201 = call "Get_Wavelength_Step.vi"("error in (no error)"=w317, ".NET Reference in"=w315) -> ("error out"=w318:errorcluster, "wavestep out"=→"Wavelength step":dbl, ".NET Reference out"=w319:refnum<k24>)  [unwired: 7 in]
            n202 = local read "Target"() -> (w301:enum32{"rdo550", "rdo570"})
            n203 = call "Get_Trigger_Step.vi"("error in (no error)"=w318, ".NET Reference in"=w319) -> ("error out"=w303:errorcluster, "triggerstep"=→"Trigger step":dbl, "Reference out"=w302:refnum<k24>)  [unwired: 7 in]
            n204 = case shown="\"rdo570\"" w301 {
              tunnel: w303 -> [_ w335]
              tunnel: w302 -> [_ w334]
              frame "rdo550", Default {
              }
              frame "rdo570" {
                n205 = call "Get_TriggerOutput_Source.vi"("error in (no error)"=w335, ".NET Reference in"=w334) -> ("mode"=→"Trigger Source":enum16{"Wavelength", "Time", ""})  [unwired: 7 in, 2 out]
              }
            }
          }
          frame "Btn_Waiting" {
            # "// Waititng for sweep status"
            n206 = flat-sequence {
              tunnel: [w344] -> w338
              tunnel: w336 -> [w345]
              tunnel: [w349] -> w337
              frame #0 {
                n207 = Tick Count (ms)() -> (millisecond timer value=w344:u32)
              }
              frame #1 {
                n208 = local read "TSL"() -> (w348:refnum<k24>)
                n209 = call "Waiting_Sweep_Status.vi"("error in (no error)"=w345, "status"="Status", "Wait time(msec)"="Wait time(msec)", ".NET Reference in"=w348) -> ()  [unwired: 6 in, 2 out]
              }
              frame #2 {
                n210 = Tick Count (ms)() -> (millisecond timer value=w349:u32)
              }
            }
            n211 = Subtract(x=w337, y=w338) -> (x-y=w339:u32)
            n212 = Number To Decimal String(number=w339) -> (decimal integer string=w342:string)  [unwired: 1 in]
            n213 = Concatenate Strings("waiting time:", w342, "msec") -> (w340:string)
            n214 = One Button Dialog(message=w340) -> ()  [unwired: 1 in, 1 out]
          }
          frame "Btn_Status" {
            # "// Get Sweep status"
            n215 = local read "TSL"() -> (w352:refnum<k24>)
            n216 = call "Get_Sweep_Status.vi"("error in (no error)"=w351, ".NET Reference in"=w352) -> ("status"=→"txtg_sweep_su":i32)  [unwired: 7 in, 2 out]
          }
          frame "Btn_GetLogg" {
            # "// Get Sweep Loggdata"
            n217 = local read "TSL"() -> (w355:refnum<k24>)
            n218 = call "Get_Logging_Data.vi"("error in (no error)"=w354, ".NET Reference in"=w355) -> ("data out"=w353:dbl[])  [unwired: 6 in, 3 out]
            n219 = call-poly <vilib>:"Write To Spreadsheet File.vi"("transpose? (no:F)"=TRUE, "1D data"=w353) -> ()  [unwired: 6 in, 1 out]
          }
          frame "Btn_Current" {
            # "// Get current cycles"
            n220 = local read "TSL"() -> (w359:refnum<k24>)
            n221 = call "Get_Sweep_Count.vi"("error in (no error)"=w357, ".NET Reference in"=w359) -> ("count out"=→"txtcurrentc":i32)  [unwired: 7 in, 2 out]
          }
          frame "Btn_Minstep" {
            # "Calucrate Minimum trigger step from sweep speed"
            n222 = local read "TSL"() -> (w361:refnum<k24>)
            n223 = call "Cal_MinimumTriggerStep_from_SweepSpeed.vi"("error in (no error)"=w360, "speed"="txtspeed", ".NET Reference in"=w361) -> ("triggerstep out"=w362:dbl)  [unwired: 6 in, 2 out]
            n224 = Number To Fractional String(number=w362) -> (F-format string=w364:string)  [unwired: 3 in]
            n225 = Concatenate Strings("Minimum trigger step = ", w364, "nm") -> (w365:string)
            n226 = One Button Dialog(message=w365) -> ()  [unwired: 1 in, 1 out]
          }
          frame "Btn_Start" {
            # "// Sweep Start"
            n227 = local read "TSL"() -> (w369:refnum<k24>)
            n228 = call "Sweep_Start.vi"("error in (no error)"=w368, ".NET Reference in"=w369) -> ()  [unwired: 8 in, 2 out]
          }
          frame "Btn_Pause" {
            # "// Sweep Pause"
            n229 = local read "TSL"() -> (w371:refnum<k24>)
            n230 = call "Sweep_Pause.vi"("error in (no error)"=w370, ".NET Reference in"=w371) -> ()  [unwired: 8 in, 2 out]
          }
          frame "Btn_ReStart" {
            # "// Sweep Restart"
            n231 = local read "TSL"() -> (w373:refnum<k24>)
            n232 = call "Sweep_Restart.vi"("error in (no error)"=w372, ".NET Reference in"=w373) -> ()  [unwired: 8 in, 2 out]
          }
          frame "Btn_Stop" {
            # "// Sweep Stop"
            n233 = local read "TSL"() -> (w375:refnum<k24>)
            n234 = call "Sweep_Pause.vi"("error in (no error)"=w374, ".NET Reference in"=w375) -> ("error out"=w376:errorcluster, "Reference out"=w377:refnum<k24>)  [unwired: 8 in]
            n235 = call "Sweep_Stop.vi"("error in (no error)"=w376, ".NET Reference in"=w377) -> ()  [unwired: 8 in, 2 out]
          }
          frame "Btn_SoftwareTrigger" {
            # "// software trigger"
            n236 = local read "TSL"() -> (w379:refnum<k24>)
            n237 = call "Set_Software_Trigger.vi"("error in (no error)"=w378, ".NET Reference in"=w379) -> ()  [unwired: 8 in, 2 out]
          }
          frame "Get IP Address" {
            n238 = local read "TSL"() -> (w382:refnum<k24>)
            n239 = call "Get_IPAddress.vi"("error in (no error)"=w380, ".NET Reference in"=w382) -> ("address"=→"IP Address":string)  [unwired: 7 in, 2 out]
          }
          frame "Get LAN Port" {
            n240 = local read "TSL"() -> (w385:refnum<k24>)
            n241 = call "Get_LAN_Portnumber.vi"("error in (no error)"=w383, ".NET Reference in"=w385) -> ("portnum"=→"LAN Port number":i32)  [unwired: 7 in, 2 out]
          }
          frame "Communication" {
            n242 = local read "Communication"() -> (w386:T2)
            n243 = case shown="\"rdiNI488\", 默认" w386 {
              frame "rdiNI488", Default {
                w387 = T7."Enabled" ("禁用")
                n244 = property on="rdiCrLf" class="Bool (严格)"("DisabledEnum"=w387) -> ()  [unwired: 2 in, 2 out]
                n245 = property on="rdiLf" class="Bool (严格)"("DisabledEnum"=w387) -> ()  [unwired: 2 in, 2 out]
              }
              frame "rdiLAN" {
                w388 = T7."Disabled and Grayed Out" ("禁用")
                n246 = local write "Port number"(5000.0 ("Port number")) -> ()
                n247 = property on="rdiCr" class="Bool (严格)"("Key Focus"=TRUE ("键选中")) -> ()  [unwired: 2 in, 2 out]
                n248 = property on="rdiLf" class="Bool (严格)"("DisabledEnum"=w388) -> ()  [unwired: 2 in, 2 out]
                n249 = property on="rdiCrLf" class="Bool (严格)"("DisabledEnum"=w388) -> ()  [unwired: 2 in, 2 out]
              }
              frame "rdiUSB" {
                w391 = T7."Disabled and Grayed Out" ("禁用")
                n250 = local read "USB device number"() -> (w393:string)
                n251 = local write "Port number"(5000.0 ("Port number")) -> ()
                n252 = local write "Address/Device number"(w393) -> ()
                n253 = property on="rdiCr" class="Bool (严格)"("Key Focus"=TRUE ("键选中")) -> ()  [unwired: 2 in, 2 out]
                n254 = property on="rdiCrLf" class="Bool (严格)"("DisabledEnum"=w391) -> ()  [unwired: 2 in, 2 out]
                n255 = property on="rdiLf" class="Bool (严格)"("DisabledEnum"=w391) -> ()  [unwired: 2 in, 2 out]
              }
            }
          }
        }
      }
      frame Error {
      }
    }
  }
  n256 = while {
    tunnel: w1 -> [w401]
    shift-right: [w397] -> w5
    shift-left: w6 -> [w396]
    stop <- w398 stop-if-true
    n257 = event shown="[41] \"Btn_Other\": 值改变" {
      selector: _ -> [_ _ _ _ _ _ _ _ _ _ _ _ _ _ _ _ _ _ _ _ _ _ _ _ _ _ _ _ _ _ _ _ _ _ _ _ _ _ _ _ _ _ _ _ _ _ _ _ _ _ _ _ _ _ _ _ _]
      dyn-events: _ -> [_ _ _ _ _ _ _ _ _ _ _ _ _ _ _ _ _ _ _ _ _ _ _ _ _ _ _ _ _ _ _ _ _ _ _ _ _ _ _ _ _ _ _ _ _ _ _ _ _ _ _ _ _ _ _ _ _]
      timeout: _ -> [_ _ _ _ _ _ _ _ _ _ _ _ _ _ _ _ _ _ _ _ _ _ _ _ _ _ _ _ _ _ _ _ _ _ _ _ _ _ _ _ _ _ _ _ _ _ _ _ _ _ _ _ _ _ _ _ _]
      tunnel: w401 -> [w406 w411 w415 w418 w423 w428 w432 w434 w439 w442 w446 w450 w454 w458 w462 w466 w470 w474 w478 w482 w486 w490 w494 w498 w502 w506 w510 w514 w518 w522 w526 w530 w534 w538 w542 w546 w550 w554 w558 w562 w566 w570 w574 w578 w582 w586 w590 w594 w598 w602 w606 _ w611 w615 w619 w623 w627]
      tunnel: w396 -> [w405 w410 w414 w417 w422 w427 w431 w433 w438 w443 w447 w449 w453 w457 w461 w465 w469 w473 w477 w481 w485 w489 w493 w497 w501 w505 w509 w513 w517 w521 w525 w529 w533 w537 w541 w545 w549 w553 w557 w561 w565 w569 w573 w577 w581 w585 w589 w593 w597 w601 w605 _ w610 w614 w618 w622 w626]
      tunnel: [w404 w409 w412 w416 w420 w425 w429 w435 w437 w441 w445 w451 w455 w459 w463 w467 w471 w475 w479 w483 w487 w491 w495 w499 w503 w507 w511 w515 w519 w523 w527 w531 w535 w539 w543 w547 w551 w555 w559 w563 w567 w571 w575 w579 w583 w587 w591 w595 w599 w603 w607 _ w612 w616 w620 w624 w628] -> w397
      tunnel: [FALSE ("stop") FALSE ("stop") _ _ w421 _ _ _ _ _ _ _ _ _ _ _ _ _ _ _ _ _ _ _ _ _ _ _ _ _ _ _ _ _ _ _ _ _ _ _ _ _ _ _ _ _ _ _ _ _ _ TRUE ("timed out?") _ _ _ _ _] -> w399
      event "Btn_Connect": Value Change {
        n258 = event-data() -> ()  [unwired: 1 in, 1 out]
        n259 = Enqueue Element(queue=w406, element="Btn_Connect" ("元素"), error in (no error)=w405) -> (error out=w404:errorcluster)  [unwired: 1 in, 2 out]
      }
      event "btnSplit": Value Change {
        n260 = event-data() -> ()  [unwired: 1 in, 1 out]
        n261 = Enqueue Element(queue=w411, element="btnSplit" ("元素"), error in (no error)=w410) -> (error out=w409:errorcluster)  [unwired: 1 in, 2 out]
      }
      event "btnGet_Visa": Value Change {
        n262 = event-data() -> ()  [unwired: 1 in, 1 out]
        n263 = Enqueue Element(queue=w415, element="btnGet_Visa" ("元素"), error in (no error)=w414) -> (error out=w412:errorcluster)  [unwired: 1 in, 2 out]
      }
      event "btnUsb_resouce": Value Change {
        n264 = event-data() -> ()  [unwired: 1 in, 1 out]
        n265 = Enqueue Element(queue=w418, element="btnUsb_resouce" ("元素"), error in (no error)=w417) -> (error out=w416:errorcluster)  [unwired: 1 in, 2 out]
      }
      event "Usb resouce": Value Change {
        n266 = event-data() -> ()  [unwired: 1 in, 1 out]
        n267 = Enqueue Element(queue=w423, element="Usbresouce_Select" ("元素"), error in (no error)=w422) -> (timed out?=w421:bool, error out=w420:errorcluster)  [unwired: 1 in, 1 out]
      }
      event "Get IP Address": Value Change {
        n268 = event-data() -> ()  [unwired: 1 in, 1 out]
        n269 = Enqueue Element(queue=w428, element="Get IP Address" ("元素"), error in (no error)=w427) -> (error out=w425:errorcluster)  [unwired: 1 in, 2 out]
      }
      event "Get LAN Port": Value Change {
        n270 = event-data() -> ()  [unwired: 1 in, 1 out]
        n271 = Enqueue Element(queue=w432, element="Get LAN Port" ("元素"), error in (no error)=w431) -> (error out=w429:errorcluster)  [unwired: 1 in, 2 out]
      }
      event "Btn_DisConnect": Value Change {
        n272 = event-data() -> ()  [unwired: 1 in, 1 out]
        n273 = Enqueue Element(queue=w434, element="Btn_DisConnect" ("元素"), error in (no error)=w433) -> (error out=w435:errorcluster)  [unwired: 1 in, 2 out]
      }
      event "BtnLD_ON": Value Change {
        n274 = event-data() -> ()  [unwired: 1 in, 1 out]
        n275 = Enqueue Element(queue=w439, element="BtnLD_ON" ("元素"), error in (no error)=w438) -> (error out=w437:errorcluster)  [unwired: 1 in, 2 out]
      }
      event "BtnLD_OFF": Value Change {
        n276 = event-data() -> ()  [unwired: 1 in, 1 out]
        n277 = Enqueue Element(queue=w442, element="BtnLD_OFF" ("元素"), error in (no error)=w443) -> (error out=w441:errorcluster)  [unwired: 1 in, 2 out]
      }
      event "BtnCoh_ON": Value Change {
        n278 = event-data() -> ()  [unwired: 1 in, 1 out]
        n279 = Enqueue Element(queue=w446, element="BtnCoh_ON" ("元素"), error in (no error)=w447) -> (error out=w445:errorcluster)  [unwired: 1 in, 2 out]
      }
      event "BtnCoh_OFF": Value Change {
        n280 = event-data() -> ()  [unwired: 1 in, 1 out]
        n281 = Enqueue Element(queue=w450, element="BtnCoh_OFF" ("元素"), error in (no error)=w449) -> (error out=w451:errorcluster)  [unwired: 1 in, 2 out]
      }
      event "BtnShutter_Open": Value Change {
        n282 = event-data() -> ()  [unwired: 1 in, 1 out]
        n283 = Enqueue Element(queue=w454, element="BtnShutter_Open" ("元素"), error in (no error)=w453) -> (error out=w455:errorcluster)  [unwired: 1 in, 2 out]
      }
      event "BtnShutter_Close": Value Change {
        n284 = event-data() -> ()  [unwired: 1 in, 1 out]
        n285 = Enqueue Element(queue=w458, element="BtnShutter_Close" ("元素"), error in (no error)=w457) -> (error out=w459:errorcluster)  [unwired: 1 in, 2 out]
      }
      event "BtnAPC": Value Change {
        n286 = event-data() -> ()  [unwired: 1 in, 1 out]
        n287 = Enqueue Element(queue=w462, element="BtnAPC" ("元素"), error in (no error)=w461) -> (error out=w463:errorcluster)  [unwired: 1 in, 2 out]
      }
      event "BtnACC": Value Change {
        n288 = event-data() -> ()  [unwired: 1 in, 1 out]
        n289 = Enqueue Element(queue=w466, element="BtnACC" ("元素"), error in (no error)=w465) -> (error out=w467:errorcluster)  [unwired: 1 in, 2 out]
      }
      event "BtndBm": Value Change {
        n290 = event-data() -> ()  [unwired: 1 in, 1 out]
        n291 = Enqueue Element(queue=w470, element="BtndBm" ("元素"), error in (no error)=w469) -> (error out=w471:errorcluster)  [unwired: 1 in, 2 out]
      }
      event "BtnmW": Value Change {
        n292 = event-data() -> ()  [unwired: 1 in, 1 out]
        n293 = Enqueue Element(queue=w474, element="BtnmW" ("元素"), error in (no error)=w473) -> (error out=w475:errorcluster)  [unwired: 1 in, 2 out]
      }
      event "Btn_SetATT": Value Change {
        n294 = event-data() -> ()  [unwired: 1 in, 1 out]
        n295 = Enqueue Element(queue=w478, element="Btn_SetATT" ("元素"), error in (no error)=w477) -> (error out=w479:errorcluster)  [unwired: 1 in, 2 out]
      }
      event "Btn_SetdBm": Value Change {
        n296 = event-data() -> ()  [unwired: 1 in, 1 out]
        n297 = Enqueue Element(queue=w482, element="Btn_SetdBm" ("元素"), error in (no error)=w481) -> (error out=w483:errorcluster)  [unwired: 1 in, 2 out]
      }
      event "Btn_SetmW": Value Change {
        n298 = event-data() -> ()  [unwired: 1 in, 1 out]
        n299 = Enqueue Element(queue=w486, element="Btn_SetmW" ("元素"), error in (no error)=w485) -> (error out=w487:errorcluster)  [unwired: 1 in, 2 out]
      }
      event "Btn_SetWavelength": Value Change {
        n300 = event-data() -> ()  [unwired: 1 in, 1 out]
        n301 = Enqueue Element(queue=w490, element="Btn_SetWavelength" ("元素"), error in (no error)=w489) -> (error out=w491:errorcluster)  [unwired: 1 in, 2 out]
      }
      event "Btn_SetFrequency": Value Change {
        n302 = event-data() -> ()  [unwired: 1 in, 1 out]
        n303 = Enqueue Element(queue=w494, element="Btn_SetFrequency" ("元素"), error in (no error)=w493) -> (error out=w495:errorcluster)  [unwired: 1 in, 2 out]
      }
      event "Btn_SetFinetuning": Value Change {
        n304 = event-data() -> ()  [unwired: 1 in, 1 out]
        n305 = Enqueue Element(queue=w498, element="Btn_SetFinetuning" ("元素"), error in (no error)=w497) -> (error out=w499:errorcluster)  [unwired: 1 in, 2 out]
      }
      event "Btn_Wavelength": Value Change {
        n306 = event-data() -> ()  [unwired: 1 in, 1 out]
        n307 = Enqueue Element(queue=w502, element="Btn_Wavelength" ("元素"), error in (no error)=w501) -> (error out=w503:errorcluster)  [unwired: 1 in, 2 out]
      }
      event "Btn_Frequency": Value Change {
        n308 = event-data() -> ()  [unwired: 1 in, 1 out]
        n309 = Enqueue Element(queue=w506, element="Btn_Frequency" ("元素"), error in (no error)=w505) -> (error out=w507:errorcluster)  [unwired: 1 in, 2 out]
      }
      event "Btn_Fine": Value Change {
        n310 = event-data() -> ()  [unwired: 1 in, 1 out]
        n311 = Enqueue Element(queue=w510, element="Btn_Fine" ("元素"), error in (no error)=w509) -> (error out=w511:errorcluster)  [unwired: 1 in, 2 out]
      }
      event "Btn_Busy": Value Change {
        n312 = event-data() -> ()  [unwired: 1 in, 1 out]
        n313 = Enqueue Element(queue=w514, element="Btn_Busy" ("元素"), error in (no error)=w513) -> (error out=w515:errorcluster)  [unwired: 1 in, 2 out]
      }
      event "Btn_Stangby": Value Change {
        n314 = event-data() -> ()  [unwired: 1 in, 1 out]
        n315 = Enqueue Element(queue=w518, element="Btn_Stangby" ("元素"), error in (no error)=w517) -> (error out=w519:errorcluster)  [unwired: 1 in, 2 out]
      }
      event "Btn_error": Value Change {
        n316 = event-data() -> ()  [unwired: 1 in, 1 out]
        n317 = Enqueue Element(queue=w522, element="Btn_error" ("元素"), error in (no error)=w521) -> (error out=w523:errorcluster)  [unwired: 1 in, 2 out]
      }
      event "Btn_GetLD": Value Change {
        n318 = event-data() -> ()  [unwired: 1 in, 1 out]
        n319 = Enqueue Element(queue=w526, element="Btn_GetLD" ("元素"), error in (no error)=w525) -> (error out=w527:errorcluster)  [unwired: 1 in, 2 out]
      }
      event "BtnPower_mode": Value Change {
        n320 = event-data() -> ()  [unwired: 1 in, 1 out]
        n321 = Enqueue Element(queue=w530, element="BtnPower_mode" ("元素"), error in (no error)=w529) -> (error out=w531:errorcluster)  [unwired: 1 in, 2 out]
      }
      event "BtnCoh_Status": Value Change {
        n322 = event-data() -> ()  [unwired: 1 in, 1 out]
        n323 = Enqueue Element(queue=w534, element="BtnCoh_Status" ("元素"), error in (no error)=w533) -> (error out=w535:errorcluster)  [unwired: 1 in, 2 out]
      }
      event "BtnShutter_Status": Value Change {
        n324 = event-data() -> ()  [unwired: 1 in, 1 out]
        n325 = Enqueue Element(queue=w538, element="BtnShutter_Status" ("元素"), error in (no error)=w537) -> (error out=w539:errorcluster)  [unwired: 1 in, 2 out]
      }
      event "BtnUnit": Value Change {
        n326 = event-data() -> ()  [unwired: 1 in, 1 out]
        n327 = Enqueue Element(queue=w542, element="BtnUnit" ("元素"), error in (no error)=w541) -> (error out=w543:errorcluster)  [unwired: 1 in, 2 out]
      }
      event "BtnAtt_value": Value Change {
        n328 = event-data() -> ()  [unwired: 1 in, 1 out]
        n329 = Enqueue Element(queue=w546, element="BtnAtt_value" ("元素"), error in (no error)=w545) -> (error out=w547:errorcluster)  [unwired: 1 in, 2 out]
      }
      event "BtnPower_dBm": Value Change {
        n330 = event-data() -> ()  [unwired: 1 in, 1 out]
        n331 = Enqueue Element(queue=w550, element="BtnPower_dBm" ("元素"), error in (no error)=w549) -> (error out=w551:errorcluster)  [unwired: 1 in, 2 out]
      }
      event "BtnPower_mW": Value Change {
        n332 = event-data() -> ()  [unwired: 1 in, 1 out]
        n333 = Enqueue Element(queue=w554, element="BtnPower_mW" ("元素"), error in (no error)=w553) -> (error out=w555:errorcluster)  [unwired: 1 in, 2 out]
      }
      event "Btnmonitor_dBm": Value Change {
        n334 = event-data() -> ()  [unwired: 1 in, 1 out]
        n335 = Enqueue Element(queue=w558, element="Btnmonitor_dBm" ("元素"), error in (no error)=w557) -> (error out=w559:errorcluster)  [unwired: 1 in, 2 out]
      }
      event "Btnmonitor_mW": Value Change {
        n336 = event-data() -> ()  [unwired: 1 in, 1 out]
        n337 = Enqueue Element(queue=w562, element="Btnmonitor_mW" ("元素"), error in (no error)=w561) -> (error out=w563:errorcluster)  [unwired: 1 in, 2 out]
      }
      event "Btn_SetWavelength_Parameters": Value Change {
        n338 = event-data() -> ()  [unwired: 1 in, 1 out]
        n339 = Enqueue Element(queue=w566, element="Btn_SetWavelength_Parameters" ("元素"), error in (no error)=w565) -> (error out=w567:errorcluster)  [unwired: 1 in, 2 out]
      }
      event "Btn_Other": Value Change {
        n340 = event-data() -> ()  [unwired: 1 in, 1 out]
        n341 = Enqueue Element(queue=w570, element="Btn_Other" ("元素"), error in (no error)=w569) -> (error out=w571:errorcluster)  [unwired: 1 in, 2 out]
      }
      event "BtnGet_setting": Value Change {
        n342 = event-data() -> ()  [unwired: 1 in, 1 out]
        n343 = Enqueue Element(queue=w574, element="BtnGet_setting" ("元素"), error in (no error)=w573) -> (error out=w575:errorcluster)  [unwired: 1 in, 2 out]
      }
      event "Btn_Waiting": Value Change {
        n344 = event-data() -> ()  [unwired: 1 in, 1 out]
        n345 = Enqueue Element(queue=w578, element="Btn_Waiting" ("元素"), error in (no error)=w577) -> (error out=w579:errorcluster)  [unwired: 1 in, 2 out]
      }
      event "Get speed table": Value Change {
        n346 = event-data() -> ()  [unwired: 1 in, 1 out]
        n347 = Enqueue Element(queue=w582, element="Get speed table" ("元素"), error in (no error)=w581) -> (error out=w583:errorcluster)  [unwired: 1 in, 2 out]
      }
      event "Target": Value Change {
        n348 = event-data() -> ()  [unwired: 1 in, 1 out]
        n349 = Enqueue Element(queue=w586, element="Target" ("元素"), error in (no error)=w585) -> (error out=w587:errorcluster)  [unwired: 1 in, 2 out]
      }
      event "Communication": Value Change {
        n350 = event-data() -> ()  [unwired: 1 in, 1 out]
        n351 = Enqueue Element(queue=w590, element="Communication" ("元素"), error in (no error)=w589) -> (error out=w591:errorcluster)  [unwired: 1 in, 2 out]
      }
      event "Btn_Status": Value Change {
        n352 = event-data() -> ()  [unwired: 1 in, 1 out]
        n353 = Enqueue Element(queue=w594, element="Btn_Status" ("元素"), error in (no error)=w593) -> (error out=w595:errorcluster)  [unwired: 1 in, 2 out]
      }
      event "Btn_GetLogg": Value Change {
        n354 = event-data() -> ()  [unwired: 1 in, 1 out]
        n355 = Enqueue Element(queue=w598, element="Btn_GetLogg" ("元素"), error in (no error)=w597) -> (error out=w599:errorcluster)  [unwired: 1 in, 2 out]
      }
      event "Btn_Current": Value Change {
        n356 = event-data() -> ()  [unwired: 1 in, 1 out]
        n357 = Enqueue Element(queue=w602, element="Btn_Current" ("元素"), error in (no error)=w601) -> (error out=w603:errorcluster)  [unwired: 1 in, 2 out]
      }
      event "Btn_Minstep": Value Change {
        n358 = event-data() -> ()  [unwired: 1 in, 1 out]
        n359 = Enqueue Element(queue=w606, element="Btn_Minstep" ("元素"), error in (no error)=w605) -> (error out=w607:errorcluster)  [unwired: 1 in, 2 out]
      }
      event Panel Close {
        n360 = event-data() -> ()  [unwired: 1 in, 1 out]
      }
      event "Btn_Start": Value Change {
        n361 = event-data() -> ()  [unwired: 1 in, 1 out]
        n362 = Enqueue Element(queue=w611, element="Btn_Start" ("元素"), error in (no error)=w610) -> (error out=w612:errorcluster)  [unwired: 1 in, 2 out]
      }
      event "Btn_Pause": Value Change {
        n363 = event-data() -> ()  [unwired: 1 in, 1 out]
        n364 = Enqueue Element(queue=w615, element="Btn_Pause" ("元素"), error in (no error)=w614) -> (error out=w616:errorcluster)  [unwired: 1 in, 2 out]
      }
      event "Btn_ReStart": Value Change {
        n365 = event-data() -> ()  [unwired: 1 in, 1 out]
        n366 = Enqueue Element(queue=w619, element="Btn_ReStart" ("元素"), error in (no error)=w618) -> (error out=w620:errorcluster)  [unwired: 1 in, 2 out]
      }
      event "Btn_Stop": Value Change {
        n367 = event-data() -> ()  [unwired: 1 in, 1 out]
        n368 = Enqueue Element(queue=w623, element="Btn_Stop" ("元素"), error in (no error)=w622) -> (error out=w624:errorcluster)  [unwired: 1 in, 2 out]
      }
      event "Btn_SoftwareTrigger": Value Change {
        n369 = event-data() -> ()  [unwired: 1 in, 1 out]
        n370 = Enqueue Element(queue=w627, element="Btn_SoftwareTrigger" ("元素"), error in (no error)=w626) -> (error out=w628:errorcluster)  [unwired: 1 in, 2 out]
      }
    }
    n371 = Unbundle By Name(w397) -> ("status"=w400:bool)
    n372 = Or(x=w400, y=w399) -> (x .or. y?=w398:bool)
  }
  n373 = Release Queue(queue=w1, error in (no error)=w5) -> ()  [unwired: 1 in, 3 out]
